vi "FPGA Audio Configure (SubVI).vi"(8 "error in (no error)":errorcluster, 9 "Read Rate (Hz)":dbl=10.0, 10 "Audio Sample Rate (kHz)":dbl=44101.0, 11 "Refnum in":refnum<k20>) -> (0 "error out":errorcluster, 1 "Required loop period (ms)":u32, 2 "Audio dt (ms)":dbl, 3 "Refnum out":refnum<k20>)   [LabVIEW 2021]
uses:
  <vilib>/Utility/error.llb/Error Cluster From Error Code.vi
  <vilib>/rvi/errors/niLvFpgaAdjustHostInterfaceError.vi
  <vilib>/rvi/interface/common/niFpgaWaitOnOcc.vi
  <vilib>/FPGAPlugInAG/Dynamic/niLvFpga_Run_Dynamic.vi
  <vilib>/rvi/interface/nirviReadWriteControl/nirviReadWriteControl.xnode
  <vilib>/rvi/interface/nirviMethod/nirviMethod.xnode
  <vilib>/rvi/errors/niLvFpgaMergeErrorWithErrorCode.vi
  NiFpgaLv.dll
  <vilib>/rvi/interface/Simulation/niFpgaSimulationCallBeginRW.vi
  <vilib>/FPGAPlugInAG/Dynamic/niLvFpga_ConfigureFifo_Dynamic.vi
  <vilib>/FPGAPlugInAG/Dynamic/niLvFpga_StartFifo_Dynamic.vi
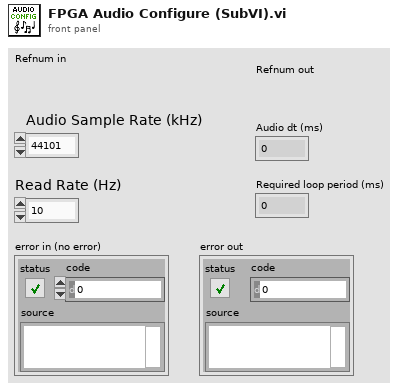
[diagram p1: front panel]
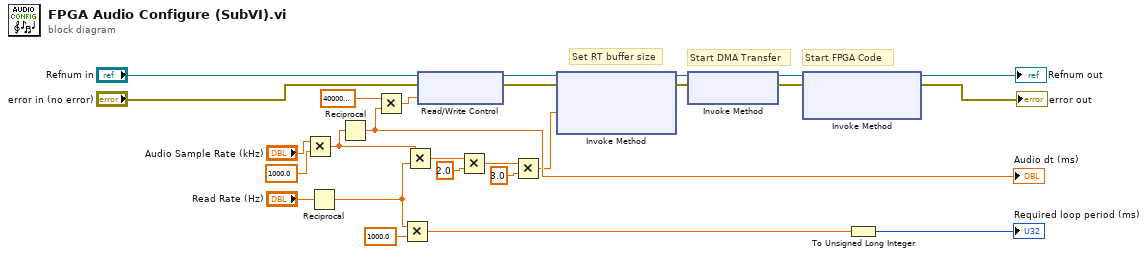
[diagram p0: block diagram]
diagram:
  # "Start FPGA Code"
  # "Start DMA Transfer"
  # "Set RT buffer size"
  n1 = Multiply(x="Audio Sample Rate (kHz)", y=1000.0) -> (x*y=w1:dbl)
  n2 = Reciprocal(x="Read Rate (Hz)") -> (1/x=w13:dbl)
  n3 = Reciprocal(x=w1) -> (1/x=w25:dbl)
  "Audio dt (ms)" <- w25
  n4 = Multiply(x=40000000.0 ("y"), y=w25) -> (x*y=w24:dbl)
  n5 = Multiply(x=w13, y=1000.0) -> (x*y=w12:dbl)
  n6 = Multiply(x=w1, y=w13) -> (x*y=w14:dbl)
  n7 = xnode "Read/Write Control"("FPGA VI Reference In"="Refnum in", "error in"="error in (no error)", "Count(Ticks)"=w24) -> ("FPGA VI Reference Out"=w22:refnum<k20>, "error out"=w20:errorcluster)
  n8 = Multiply(x=w14, y=2.0) -> (x*y=w16:dbl)
  n9 = Multiply(x=w16, y=3.0) -> (x*y=w18:dbl)
  n10 = xnode "Invoke Method"("FPGA VI Reference In"=w22, "error in"=w20, "Requested Depth"=w18) -> ("FPGA VI Reference Out"=w4:refnum<k20>, "error out"=w9:errorcluster)  [unwired: 1 out]
  n11 = xnode "Invoke Method"("FPGA VI Reference In"=w4, "error in"=w9) -> ("FPGA VI Reference Out"=w6:refnum<k20>, "error out"=w7:errorcluster)
  n12 = xnode "Invoke Method"("FPGA VI Reference In"=w6, "error in"=w7) -> ("FPGA VI Reference Out"=→"Refnum out":refnum<k20>, "error out"=→"error out":errorcluster)  [unwired: 1 in]
  n13 = To Unsigned Long Integer(number=w12) -> (unsigned 32bit integer=→"Required loop period (ms)":u32)
